vi "XOR Tester.vi"() -> ()   [LabVIEW 2015, in "Neural Network.lvclass"]
uses:
  Neural Network/Neural Network.lvclass
  Neural Network/Types/Teaching Settings.ctl
  <vilib>/Math Plots/3D Math Plots/3D Surface/3D Surface XCtrl/3D Surface.xctl
panel:
  out "Response Surface Output 0":refnum<class "3D Plot Datatype.lvclass">[](xcontrol)
  out "Teaching Time (s)":dbl=0.043538570404052734
  out "Response Surface Output 1":refnum<class "3D Plot Datatype.lvclass">[](xcontrol)
  out "Goal Reached":bool=TRUE
  out "Error Trend":dbl[][](graph)=[[1.3012234148046902, 1.1767554614349676, 1.0149523475504416, 0.8108670892383649, 0.8102279943111259, 0.9111041804384064, 1.0315038165335366, 1.0311729978237232, 0.9709948112599156, 0.8974401996661905, 0.8971292555679361, 0.9331874100014973, 0.9730579639160948, 0.9709163533021855, 0.9486096054703024, 0.924570234400466, 0.9253337418747704, 0.9382861302417811, 0.9416085275445258, 0.9371942712020436, 0.9383493719425021, 0.9395972473940272, 0.9397442665803076, 0.9415974810614813, 0.9475006824505275, 0.9413648126196477, 0.9283157825113576, 0.9286182362581612, 0.9355628040534726, 0.9417579707594679, 0.9438147500347812, 0.9408981519385695, 0.9361945422361803, 0.9319308103307764, 0.9322220768014736, 0.9329476845483253, 0.935555000523162, 0.9355562882673899, 0.9343606219681202, 0.933607909019378, 0.933055388045709, 0.9326412246337776, 0.9339409903419675, 0.9349091124983308, 0.9322136983144376, 0.9286970019760297, 0.9250379377057035, 0.9219742116395568, 0.9160086430073742, 0.9092694293418273, 0.910903337787796, 0.90897893982547, 0.9068790340403168, 0.9043381666187567, 0.9022369953747049, 0.9018907397841931, 0.900502679016288, 0.8852464220424523, 0.8727819701777081, 0.8581216032758914, 0.8342380691576199, 0.8093759706962207, 0.7809780216586786, 0.7451667467162603, 0.703554706886707, 0.6579593772727416, 0.6558374319675913, 0.6573107736007149, 0.6885140448461757, 0.6627392415077731, 0.6572792158965804, 0.6625799266011103, 0.6384598440570773, 0.6695353020661046, 0.6598852837868343, 0.6225124304283375, 0.6362950401373193, 0.6364226163064413, 0.6259691358969846, 0.632532577076899, 0.6243673779593264, 0.6124317100690793, 0.6122140616852386, 0.6262757535850919, 0.610234708131659, 0.5836047297153354, 0.5767681168453287, 0.5730750379849154, 0.5820719624308494, 0.5812990956885722, 0.5822809322725857, 0.5812423328413696, 0.5776724194093755, 0.5826793469215125, 0.58344153686843, 0.5788910865922986, 0.5714662402970638, 0.5684790232926216, 0.5645725534028018, 0.5598010451731196, 0.554178956917992, 0.5478699069333676, 0.5367850578864143, 0.4960038035913762, 0.2776048542743103, 0.178362822247398, 0.16774984204863588, 0.19811450878269923, 0.20673113829018122, 0.19963104942866605, 0.20113764102683498, 0.20704215375975743, 0.21733808992928333, 0.22907968153701141, 0.20431637114026596, 0.15920023370244846, 0.137646365727541, 0.1118374026491107, 0.07587475864360285, 0.044922416395198825, 0.043424580002214656, 0.021610462184618283, 0.05128204865269551, 0.08119335354507667, 0.050725011242595854, 0.15976522135956578], [1.3175367649975172, 1.1663293057059105, 0.9703674960543722, 0.7310580646291422, 0.7325726734863046, 0.8526771418279875, 0.9993648485604227, 0.999893592861549, 0.92745983922382, 0.918939240047439, 0.9517034791785143, 0.9548973099349419, 0.9379209443528703, 0.9180180466775772, 0.9164513375347386, 0.9264028091565739, 0.9390691302261445, 0.9396988450216376, 0.9329144245146744, 0.9321397492061078, 0.9343294418816166, 0.9366757423453983, 0.935174998402577, 0.9265352427703436, 0.9057009287695188, 0.9095361677284186, 0.92625988163489, 0.9329471898943018, 0.931876274017171, 0.9310767638902063, 0.9326826802084027, 0.9391776692515499, 0.9381087796635551, 0.9366753704629079, 0.9308378271493155, 0.9329368158707366, 0.9350917837761746, 0.9357587409132211, 0.9346730484411003, 0.9325057788806674, 0.9342559572781095, 0.9346997323061732, 0.9269747274757278, 0.9226620953146756, 0.9176289451246133, 0.9104848976340436, 0.9020642255079969, 0.8928893822767892, 0.8903456787997723, 0.8818802027684004, 0.8595395107155877, 0.8416294885830432, 0.8218108935440189, 0.8011786401383496, 0.7800595913441158, 0.7610076650319096, 0.7429395836024429, 0.7229900594777094, 0.7023556679530667, 0.6814382470044666, 0.6683252086940156, 0.6605896137410187, 0.6562094648768944, 0.6508792658980552, 0.6463407433823101, 0.6439090798814346, 0.6452334481016337, 0.6409101566289642, 0.647826855510374, 0.6395848349329059, 0.6398810117845432, 0.6329705529067204, 0.6215958394692709, 0.6333627534186098, 0.637449222434049, 0.6348747459783409, 0.6365608920043314, 0.6339712043794592, 0.6263812045805446, 0.6255762070175417, 0.6261350012123317, 0.6259525210638418, 0.6294693690911498, 0.631185949538329, 0.628720884292617, 0.6274318218269651, 0.6275097688070121, 0.6274316550664576, 0.6231784794606579, 0.6268624752127135, 0.6333565804997473, 0.6322527927456584, 0.6290500874784746, 0.6280852463198909, 0.6299935380929984, 0.6332097186818519, 0.63504320333313, 0.6359384141425629, 0.6361465743072584, 0.6367151563907304, 0.6374617357690319, 0.6379621997341877, 0.638884689167856, 0.634264671800327, 0.5858037702836729, 0.562512957270953, 0.5617212721858348, 0.5641048975660614, 0.5613316238851059, 0.5555965039688658, 0.550863513178327, 0.5456782987293503, 0.5397352395133403, 0.5323008722445126, 0.5228245596542547, 0.5108961856906451, 0.49766007747181296, 0.483071326939834, 0.46615998300914707, 0.4402877418653494, 0.4432010686700046, 0.3895601964537517, 0.32053083444736724, 0.27384220902925493, 0.23442976582344052, 0.1866433947793815]]
  # "The succes rate for finding \na solution to the XOR \nproblem is smaller \nthan 100%. Sometimes you \nneed to re-run\nthe example multiple times.\n\nThe values of XOR are not 0\nand 1 to present the ability\nto scale inputs and outputs\ninside the API."
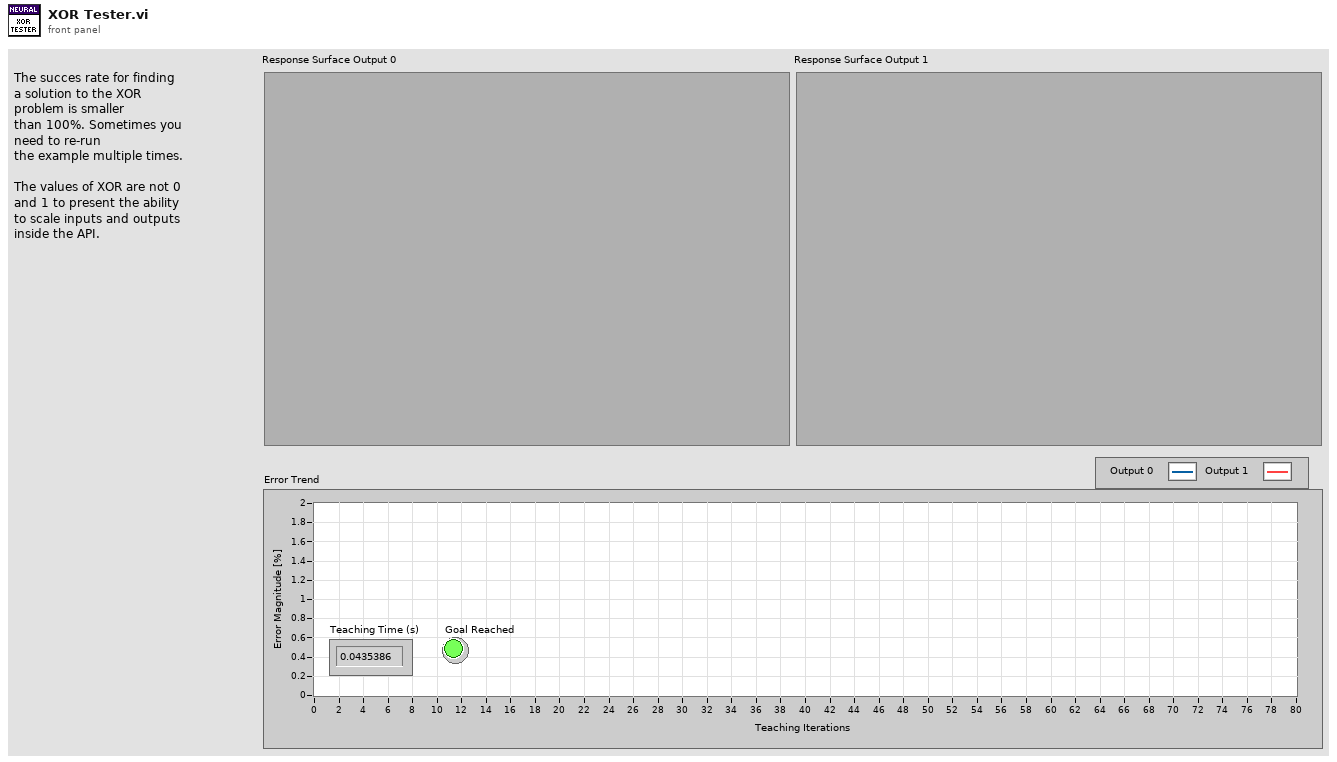
[diagram p1: front panel]
types:
  T1 = typedef "Neural Network.lvclass/Teaching Settings.ctl" = cluster{"Max Epocs":u64, "Max Time (s)":dbl, "Error Goal (%)":dbl, "# Vectors per Iteration":i64}
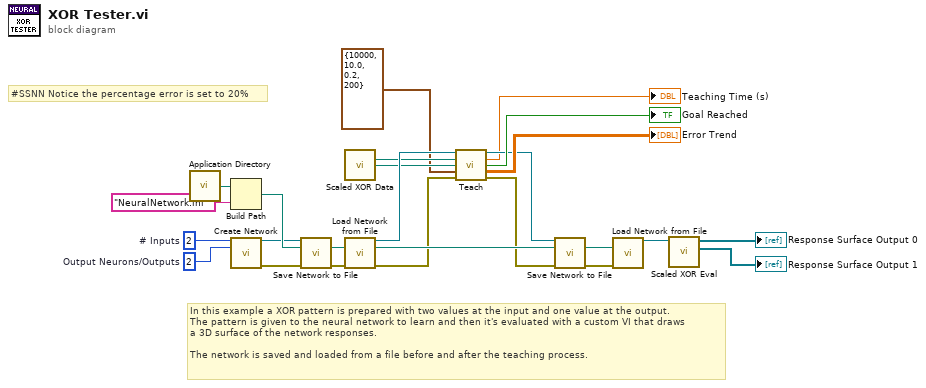
[diagram p0: block diagram]
diagram:
  w9 = u32 2  # Output Neurons/Outputs
  w10 = u32 2  # # Inputs
  # "#SSNN Notice the percentage error is set to 20%"
  # "In this example a XOR pattern is prepared with two values at the input and one value at the output.\nThe pattern is given to the neural network to learn and then it's evaluated with a custom VI that draws\na 3D surface of the network responses.\n\nThe network is saved and loaded from a file before and after the teaching process."
  n1 = call <vilib>:"Application Directory.vi"() -> ("Application Directory"=w18:path)
  n2 = Build Path(base path=w18, name or relative path="NeuralNetwork.ini") -> (appended path=w16:path)
  n3 = call "Create Network.vi"("#Inputs"=w10, "#Outputs"=w9) -> ("Neural Network"=w8:refnum<class "Neural Network.lvclass">, "Error Out"=w7:errorcluster)  [unwired: 12 in]
  n4 = call "Save Network to File.vi"("Neural Network In"=w8, "File Path (dialog)"=w16, "Error In"=w7) -> ("Path Used"=w15:path, "Error Out"=w25:errorcluster)  [unwired: 10 in, 1 out]
  n5 = call "Scaled XOR Data.vi"() -> ("XOR File Out"=w3:path, "XOR_VAL File Out"=w2:path)  [unwired: 14 in]
  n6 = call "Load Network from File.vi"("File Path (dialog)"=w15, "Error In"=w25) -> ("Neural Network Out"=w23:refnum<class "Neural Network.lvclass">, "Used Path"=w24:path, "Error Out"=w22:errorcluster)  [unwired: 10 in, 1 out]
  n7 = call "Teach.vi"("Neural Network In"=w23, "Teaching File Path"=w3, "Validation File Path"=w2, "Settings"=T1 {"Max Epocs"=10000, "Max Time (s)"=10.0, "Error Goal (%)"=0.2, "# Vectors per Iteration"=200}, "Error In"=w22) -> ("Neural Network Out"=w19:refnum<class "Neural Network.lvclass">, "Teaching Time (s)"=→"Teaching Time (s)":dbl, "Solution Found"=→"Goal Reached":bool, "% Error / Output"=→"Error Trend":dbl[][], "Error Out"=w6:errorcluster)  [unwired: 6 in]
  n8 = call "Save Network to File.vi"("Neural Network In"=w19, "File Path (dialog)"=w24, "Error In"=w6) -> ("Path Used"=w14:path, "Error Out"=w13:errorcluster)  [unwired: 10 in, 1 out]
  n9 = call "Load Network from File.vi"("File Path (dialog)"=w14, "Error In"=w13) -> ("Neural Network Out"=w11:refnum<class "Neural Network.lvclass">)  [unwired: 10 in, 3 out]
  n10 = call "Scaled XOR Eval.vi"("Neural Network Out"=w11) -> ("Output 1"=→"Response Surface Output 1":refnum<class "3D Plot Datatype.lvclass">[], "Output 0"=→"Response Surface Output 0":refnum<class "3D Plot Datatype.lvclass">[])  [unwired: 9 in]
